vi "FestoCPX.Valve(1out2in).vi"(6 "Timeout [ms] (5000)":u32=5000, 8 "error in (no error)":errorcluster, 9 "Position":T3, 10 "Output":T1, 11 "Inputs":T2[](array[typedef])) -> (0 "error out":errorcluster, 2 "Aborted?":bool, 3 "Timeout?":bool)   [LabVIEW 2016]
uses:
  Station/Station.ValvePosition.ctl
  FestoCPX.DI.Signal.ctl
  FestoCPX.DO.Signal.ctl
  FestoCPX.DO.Data.State.Set.vi
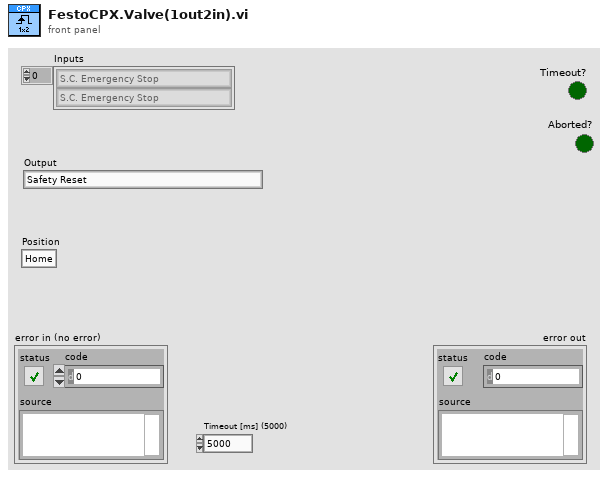
[diagram p1: front panel]
types:
  T1 = typedef "FestoCPX.DO.Signal.ctl" = enum16{"Safety Reset", "Air Main Valve", "Door Lock", "Button LED Start", "Button LED Stop", "Button LED Control", "Traffic LED Red", "Traffic LED Orange", "Traffic LED Green", "Horn", "Laser Interlock", "Laser Trigger", "Laser Fume Extractor", "Product Suction Gripper Slot 1 A", "Product Suction Gripper Slot 1 B", "Product Suction Gripper Slot 2 A", "Product Suction Gripper Slot 2 B", "Product Suction Gripper Slot 3 A", "Product Suction Gripper Slot 3 B", "Product Suction Gripper Slot 4 A", "Product Suction Gripper Slot 4 B", "Product Suction Gripper Final A", "Product Suction Gripper Final B", "Lamp", "Q1 Product Move Work", "Q1 Product Move Home", "Q2 Table Turn Work", "Q2 Table Turn Home", "Q3 Product Lift A", "Q3 Product Lift B", "Q4 Product Arm OK", "Q4 Product Arm NOK", "Q5 Product Arm Work", "Q6 Product BlowOut A", "Q6 Product BlowOut B"}
  T2 = typedef "FestoCPX.DI.Signal.ctl" = enum16{"S.C. Emergency Stop", "S.C. Side Door Close", "S.C. Front Door Close", "S.C. Front Door Secured", "Button Start", "Button Stop", "Button Control", "Product Move Home", "Product Move Work", "Table Position", "Table Lock", "Product Lift A Home", "Product Lift B Home", "Product Arm OK", "Product Arm NOK", "Product Arm Work", "Revolver ID 1", "Revolver ID 2", "Revolver ID 3", "Revolver ID 4", "Revolver ID 5", "Air Pressure Inside", "Air Pressure Inlet", "Product Slot 1 A Present", "Product Slot 1 B Present", "Product Slot 2 A Present", "Product Slot 2 B Present", "Product Slot 3 A Present", "Product Slot 3 B Present", "Product Slot 4 A Present", "Product Slot 4 B Present", "Product Final A Present", "Product Final B Present", "Product Output A Present", "Product Output B Present", "Product Container OK Present", "Product Container NOK Present", "Fork ID 1", "Fork ID 2"}
  T3 = typedef "Station.ValvePosition.ctl" = enum16{"Home", "Work"}
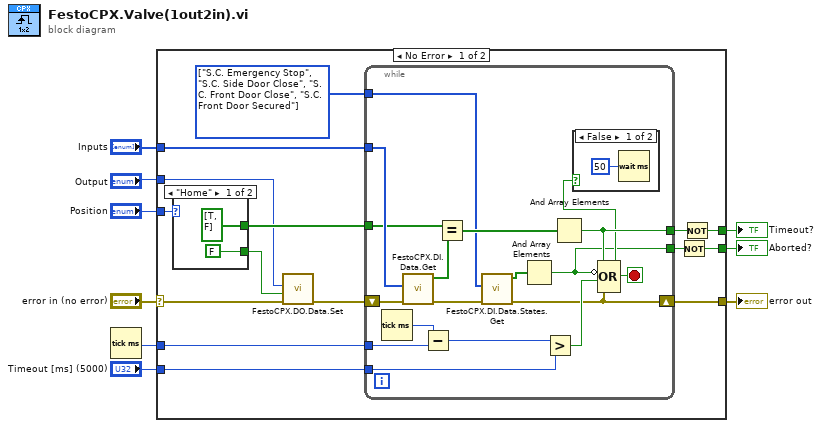
[diagram p0: block diagram]
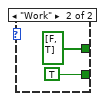
[diagram p2: hidden frame]
diagram:
  n1 = Tick Count (ms)() -> (millisecond timer value=w5:u32)
  n2 = case shown="No Error" "error in (no error)" {
    selector: "error in (no error)" -> [w18 w47]
    tunnel: "Position" -> [w17 _]
    tunnel: [w13 w47] -> w8
    tunnel: [w21 _] -> w7
    tunnel: w5 -> [w24 _]
    tunnel: "Timeout [ms] (5000)" -> [w23 _]
    tunnel: "Inputs" -> [w22 _]
    tunnel: "Output" -> [w14 _]
    tunnel: [w10 _] -> w1
    frame No Error {
      w12 = T2[] [enum."S.C. Emergency Stop", enum."S.C. Side Door Close", enum."S.C. Front Door Close", enum."S.C. Front Door Secured"] items=["S.C. Emergency Stop", "S.C. Side Door Close", "S.C. Front Door Close", "S.C. Front Door Secured", "Button Start", "Button Stop", "Button Control", "Product Move Home", "Product Move Work", "Table Position", "Table Lock", "Product Lift A Home", "Product Lift B Home", "Product Arm OK", "Product Arm NOK", "Product Arm Work", "Revolver ID 1", "Revolver ID 2", "Revolver ID 3", "Revolver ID 4", "Revolver ID 5", "Air Pressure Inside", "Air Pressure Inlet", "Product Slot 1 A Present", "Product Slot 1 B Present", "Product Slot 2 A Present", "Product Slot 2 B Present", "Product Slot 3 A Present", "Product Slot 3 B Present", "Product Slot 4 A Present", "Product Slot 4 B Present", "Product Final A Present", "Product Final B Present", "Product Output A Present", "Product Output B Present", "Product Container OK Present", "Product Container NOK Present", "Fork ID 1", "Fork ID 2"] ("CPX.DI")
      n3 = case shown="\"Home\"" w17 {
        tunnel: [bool[] [TRUE, FALSE] bool[] [FALSE, TRUE]] -> w15
        tunnel: [FALSE TRUE] -> w16
        frame "Home" {
        }
        frame "Work" {
        }
      }
      n4 = call-poly "FestoCPX.DO.Data.Set.vi"("error in (no error)"=w18, "State"=w16, "CPX.DO"=w14) -> ("error out"=w20:errorcluster)  [unwired: 8 in]
      n5 = while {
        shift-right: [w33] -> w13
        shift-left: w20 -> [w45]
        tunnel: w22 -> [w44]
        tunnel: [w36] -> w19
        tunnel: w24 -> [w42]
        tunnel: w23 -> [w40]
        tunnel: w15 -> [w39]
        tunnel: w12 -> [w32]
        tunnel: [w31] -> w11
        stop <- w35 stop-if-true
        n6 = Tick Count (ms)() -> (millisecond timer value=w43:u32)
        n7 = call-poly "FestoCPX.DI.Data.Get.vi"("error in (no error)"=w45, "CPX.DI"=w44) -> ("error out"=w34:errorcluster, "State"=w29:bool[])  [unwired: 5 in, 3 out]
        n8 = Subtract(x=w43, y=w42) -> (x-y=w41:u32)
        n9 = Equal?(x=w39, y=w29) -> (x = y?=w38:bool[])
        n10 = call "FestoCPX.DI.Data.States.Get.vi"("error in (no error)"=w34, "CPX.DI"=w32) -> ("error out"=w33:errorcluster, "State"=w30:bool[])  [unwired: 5 in, 3 out]
        n11 = And Array Elements(Boolean array=w30) -> (logical AND=w31:bool)
        n12 = Greater?(x=w41, y=w40) -> (0:w37:bool)
        n13 = And Array Elements(Boolean array=w38) -> (logical AND=w36:bool)
        n14 = Compound Arithmetic op=OR(w36, invert w31, w37, w33) -> (w35:bool)
        n15 = case shown="False" w35 {
          frame False {
            n16 = Wait (ms)(milliseconds to wait=u32 50) -> ()  [unwired: 1 out]
          }
          frame True {
          }
        }
      }
      n17 = Not(x=w11) -> (.not. x?=w10:bool)
      n18 = Not(x=w19) -> (.not. x?=w21:bool)
    }
    frame Error {
    }
  }
  "error out" <- w8
  "Timeout?" <- w7
  "Aborted?" <- w1
